vi "Script_Create Wheel.vi"(6 "error source terminal refnum":refnum<vi>, 8 "error in (no error)":errorcluster, 10 "owner diagram refnum":refnum<vi>, 11 "wheel in":refnum<class "NI_Robotics_Wheel.lvclass">) -> (0 "error out":errorcluster, 1 "created?":bool, 2 "wheel out terminal refnum":refnum<vi>, 4 "error out terminal refnum":refnum<vi>)   [LabVIEW 2017, in "NI_Robotics_Scripting Utilities.lvlib"]
uses:
  <vilib>/robotics/Utilities/Scripting/NI_Robotics_Scripting Utilities.lvlib
  <vilib>/robotics/Steering/Wheel/NI_Robotics_Wheel.lvclass
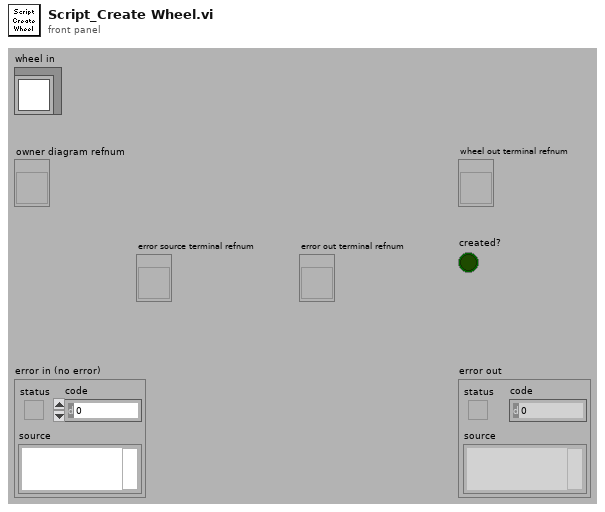
[diagram p1: front panel]
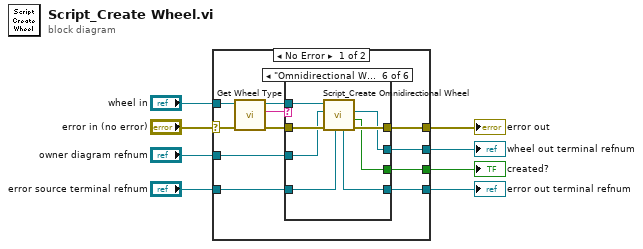
[diagram p0: block diagram]
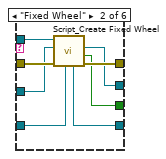
[diagram p3: hidden frame]
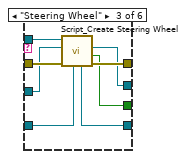
[diagram p4: hidden frame]
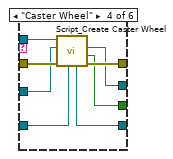
[diagram p5: hidden frame]
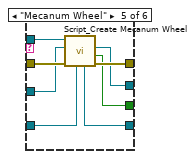
[diagram p6: hidden frame]
diagram:
  n1 = case shown="No Error" "error in (no error)" {
    selector: "error in (no error)" -> [w18 w62]
    tunnel: "wheel in" -> [w19 _]
    tunnel: "owner diagram refnum" -> [w14 _]
    tunnel: [w13 w62] -> w6
    tunnel: [w12 _] -> w4
    tunnel: [w11 _] -> w3
    tunnel: [w10 _] -> w2
    tunnel: "error source terminal refnum" -> [w9 _]
    frame No Error {
      n2 = call-dynamic "Get Wheel Type.vi"("error in (no error)"=w18, "wheel in"=w19) -> ("error out"=w15:errorcluster, "wheel type"=w17:string, "wheel out"=w16:refnum<class "NI_Robotics_Wheel.lvclass">)  [unwired: 7 in]
      n3 = case shown="\"Omnidirectional Wheel\"" w17 {
        tunnel: w16 -> [_ w29 w37 w45 w53 w61]
        tunnel: w15 -> [w21 w28 w36 w44 w52 w60]
        tunnel: w14 -> [_ w26 w35 w42 w50 w59]
        tunnel: [w21 w27 w34 w43 w51 w56] -> w13
        tunnel: [_ w25 w30 w38 w46 w54] -> w12
        tunnel: [_ w24 w31 w39 w47 w55] -> w11
        tunnel: [w20 w23 w32 w40 w48 w57] -> w10
        tunnel: w9 -> [w20 w22 w33 w41 w49 w58]
        frame Default {
        }
        frame "Fixed Wheel" {
          n4 = call <vilib>:"Script_Create Fixed Wheel.vi"("error source terminal refnum"=w22, "error in (no error)"=w28, "owner diagram refnum"=w26, "wheel in"=w29) -> ("error out"=w27:errorcluster, "created?"=w24:bool, "wheel out terminal refnum"=w25:refnum<vi>, "error out terminal refnum"=w23:refnum<vi>)  [unwired: 4 in]
        }
        frame "Steering Wheel" {
          n5 = call <vilib>:"Script_Create Steering Wheel.vi"("error source terminal refnum"=w33, "error in (no error)"=w36, "owner diagram refnum"=w35, "wheel in"=w37) -> ("error out"=w34:errorcluster, "created?"=w31:bool, "wheel out terminal refnum"=w30:refnum<vi>, "error out terminal refnum"=w32:refnum<vi>)  [unwired: 4 in]
        }
        frame "Caster Wheel" {
          n6 = call <vilib>:"Script_Create Caster Wheel.vi"("error source terminal refnum"=w41, "error in (no error)"=w44, "owner diagram refnum"=w42, "wheel in"=w45) -> ("error out"=w43:errorcluster, "created?"=w39:bool, "wheel out terminal refnum"=w38:refnum<vi>, "error out terminal refnum"=w40:refnum<vi>)  [unwired: 4 in]
        }
        frame "Mecanum Wheel" {
          n7 = call <vilib>:"Script_Create Mecanum Wheel.vi"("error source terminal refnum"=w49, "error in (no error)"=w52, "owner diagram refnum"=w50, "wheel in"=w53) -> ("error out"=w51:errorcluster, "created?"=w47:bool, "wheel out terminal refnum"=w46:refnum<vi>, "error out terminal refnum"=w48:refnum<vi>)  [unwired: 4 in]
        }
        frame "Omnidirectional Wheel" {
          n8 = call <vilib>:"Script_Create Omnidirectional Wheel.vi"("error source terminal refnum"=w58, "error in (no error)"=w60, "owner diagram refnum"=w59, "wheel in"=w61) -> ("error out"=w56:errorcluster, "created?"=w55:bool, "wheel out terminal refnum"=w54:refnum<vi>, "error out terminal refnum"=w57:refnum<vi>)  [unwired: 4 in]
        }
      }
    }
    frame Error {
    }
  }
  "error out" <- w6
  "wheel out terminal refnum" <- w4
  "created?" <- w3
  "error out terminal refnum" <- w2
